vi "Typecast.vi"(8 "error in (no error)":errorcluster, 11 "Data in":refnum<class "Data.lvclass">) -> (0 "error out":errorcluster, 3 "Data_Gaze out":refnum<class "Data_AllInOne.lvclass">)   [LabVIEW 2020, in "Data_AllInOne.lvclass"]
uses:
  Data_AllInOne.lvclass
  Data.lvclass
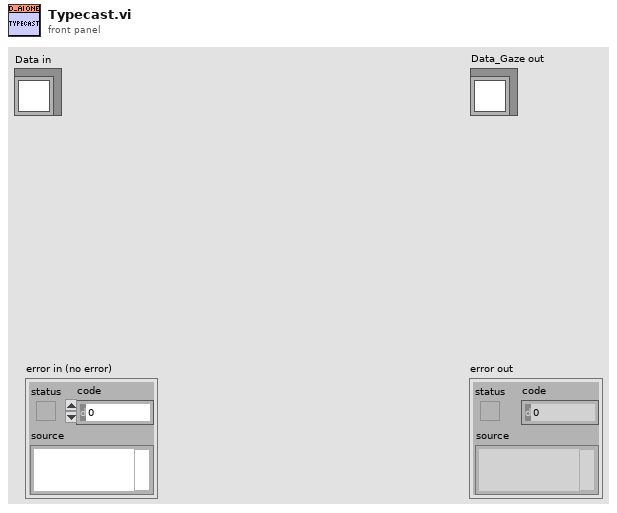
[diagram p1: front panel]
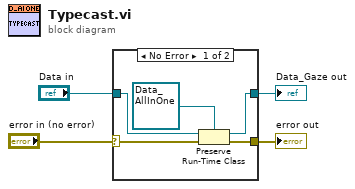
[diagram p0: block diagram]
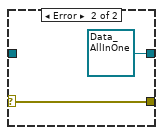
[diagram p2: hidden frame]
diagram:
  n1 = case shown="No Error" "error in (no error)" {
    selector: "error in (no error)" -> [w9 w11]
    tunnel: [w8 w11] -> w3
    tunnel: [w7 refnum<class "Data_AllInOne.lvclass"> refnum ("Data_Pupil_Diameter in")] -> w2
    tunnel: "Data in" -> [w5 _]
    frame No Error {
      n2 = Preserve Run-Time Class(object in=w5, error in=w9, 2:refnum<class "Data_AllInOne.lvclass"> refnum ("Data_Pupil_Diameter in")) -> (object out=w7:refnum<class "Data_AllInOne.lvclass">, error out=w8:errorcluster)
    }
    frame Error {
    }
  }
  "error out" <- w3
  "Data_Gaze out" <- w2
